vi "ResonanceAnalyzer.vi"() -> ()   [LabVIEW 2015]
uses:
  <vilib>/imath/engines/lvmath/Plug In/_Char/NIMS_CH_character datatype.ctl
  <vilib>/imath/engines/lvmath2/RunTimeEngine/Managers/WorkSpace/UID Generator.vi
  <vilib>/imath/engines/lvmath2/RunTimeEngine/RunTimeType/NIMS_RunTimeType_From StrictType (excl LVString).vi
  <instcachedir>/0/NIMS_RunTimeType_From StrictType (excl LVString)_EB1C38A9BC5048DA9ABDA8F781E54D21.lvgen/NIMS_RunTimeType_From StrictType (excl LVString)_EB1C38A9BC5048DA9ABDA8F781E54D21_000.vi
  <vilib>/imath/engines/lvmath2/RunTimeEngine/LocalVariableDefStatement/MC_LocalVariableDefStatement_Display.vi
  <vilib>/imath/engines/lvmath/Plug In/_Char/NIMS_CH_Character RV to String.vi
  <vilib>/imath/engines/lvmath2/RunTimeEngine/BuiltInFunctions/random/NIMS_random.vi
  <vilib>/imathl/engines/lvmath/Functions/Error Handling/Create Error.vi
  <vilib>/imath/engines/lvmath2/RunTimeEngine/NodeEndStatement/NIMS_NodeEndStatement_Get Scalar.vi
  <instcachedir>/0/NIMS_NodeEndStatement_Get Scalar_EFB59FDA1E10412DB5B4364F310E1970.lvgen/NIMS_NodeEndStatement_Get Scalar_EFB59FDA1E10412DB5B4364F310E1970_000.vi
  <vilib>/imath/engines/lvmath/Functions/Error Handling/MergeErrorsWrapper.vi
  <vilib>/imath/engines/lvmath2/RunTimeEngine/Managers/SymbolTable/Clear UID.vi
  <vilib>/imath/engines/lvmath2/RunTimeEngine/NodeEndStatement/NIMS_NodeEndStatement_Output.vi
  <instcachedir>/0/NIMS_NodeEndStatement_Output_53EC0D466D134D7ABD903AC30B43404B.lvgen/NIMS_NodeEndStatement_Output_53EC0D466D134D7ABD903AC30B43404B_001.vi
  <vilib>/imath/engines/lvmath2/RunTimeEngine/ErrorHandling/NIMS_Finalize Error.vi
  <vilib>/Utility/file.llb/Read Delimited Spreadsheet (DBL).vi
  <vilib>/imath/engines/lvmath2/RunTimeEngine/Managers/SymbolTable/NIMS_WorkSpace.lvlib
panel:
  out "XY Graph 2":cluster{"all rows":dbl[], "Array":dbl[]}(graph)
  out "Array 3":dbl[](array[numeric])
  out "Array 2":dbl[](array[numeric])
  out "Array":dbl[](array[numeric])
  out "XY Graph":cluster{"i":dbl[], "y":dbl[]}(graph)
  in  "Input Parameters":T1
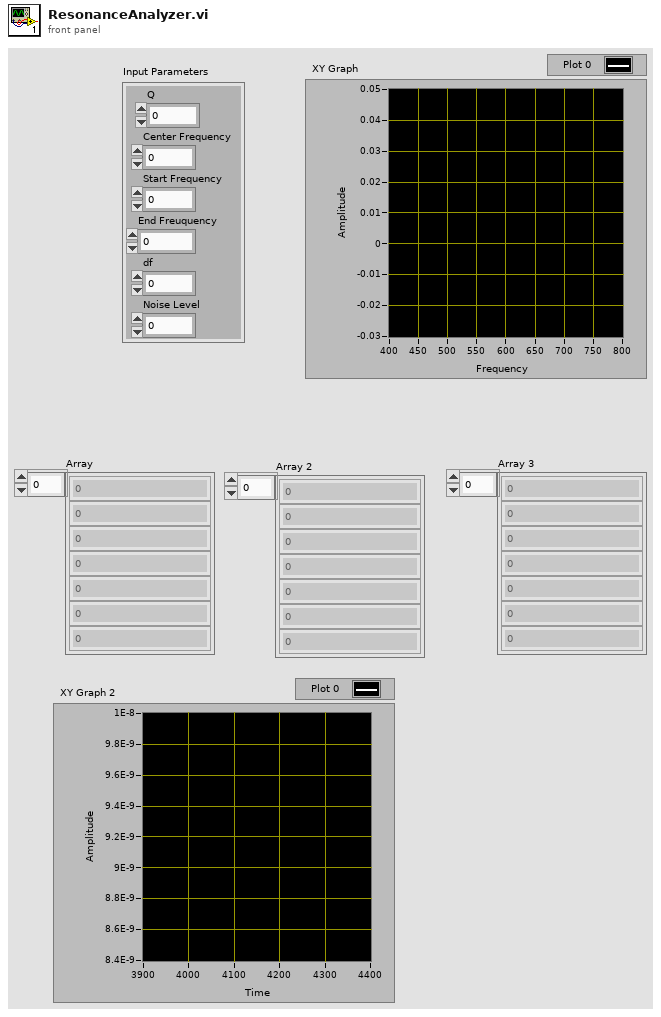
[diagram p1: front panel]
types:
  T1 = cluster{"Q":dbl, "Center Frequency ":dbl, "Start Frequency":dbl, "End Freuquency":dbl, "df":dbl, "Noise Level":dbl}
  T2 = typedef "NIMS_CH_character datatype.ctl" = cluster{"Numeric":u8}
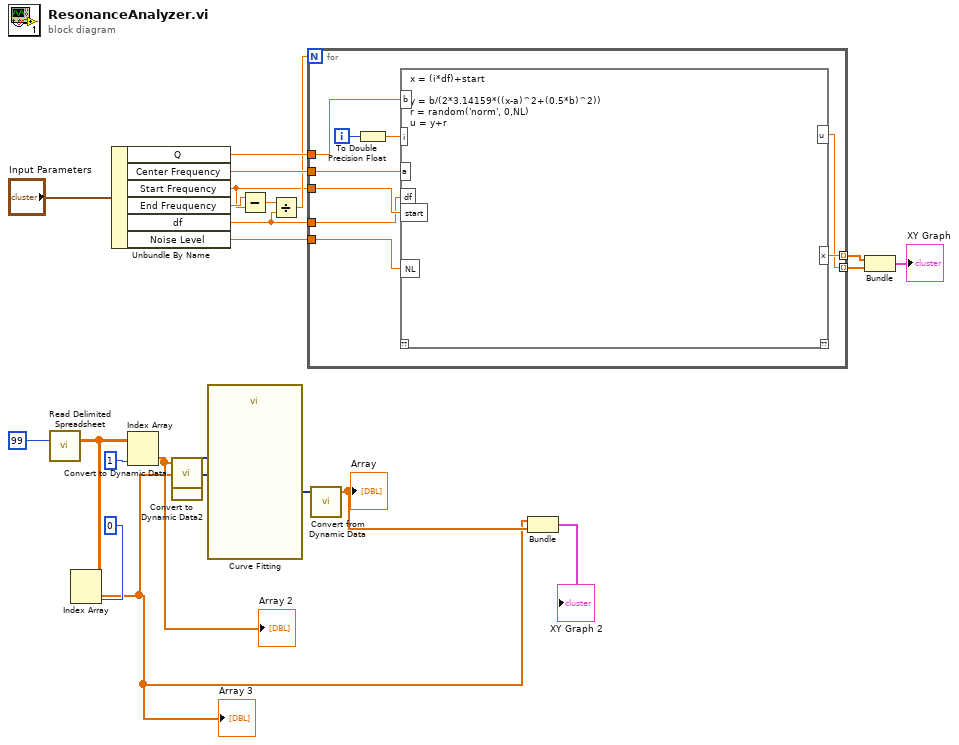
[diagram p0: block diagram]
diagram:
  n1 = call-poly <vilib>:"Read Delimited Spreadsheet.vi"("number of rows (all:-1)"=99) -> ("all rows"=w9:dbl[][])  [unwired: 9 in, 5 out]
  n2 = Index Array(array=w9, index (col)=0) -> (element=w2:dbl[])  [unwired: 1 in]
  "Array 3" <- w2
  n3 = Unbundle By Name("Input Parameters") -> ("Q"=w22:dbl, "Center Frequency"=w21:dbl, "Start Frequency"=w12:dbl, "End Freuquency"=w13:dbl, "df"=w16:dbl, "Noise Level"=w20:dbl)
  n4 = Index Array(array=w9, index (col)=1) -> (element=w6:dbl[])  [unwired: 1 in]
  "Array 2" <- w6
  n5 = call "Convert to Dynamic Data"("Array"=w6) -> ("Dynamic Data Type"=w5:dynamicdata)  [unwired: 3 in]
  n6 = call "Convert to Dynamic Data2"("Array"=w2) -> ("Dynamic Data Type"=w4:dynamicdata)  [unwired: 3 in]
  n7 = call "Curve Fitting"("Locations"=w4, "Signals"=w5) -> ("best fit"=w10:dynamicdata)  [unwired: 5 in, 4 out]
  n8 = Subtract(x=w13, y=w12) -> (x-y=w15:dbl)
  n9 = Divide(x=w15, y=w16) -> (x/y=w14:dbl)
  n10 = for {
    N: w14 -> [_]
    tunnel: [w32] -> w23 mode=indexing
    tunnel: [w31] -> w18 mode=indexing
    tunnel: w22 -> [w30]
    tunnel: w21 -> [w29]
    tunnel: w12 -> [w28]
    tunnel: w16 -> [w27]
    tunnel: w20 -> [w26]
    i -> [w25]
    n11 = To Double Precision Float(number=w25) -> (double precision float=w24:dbl)
    n12 = mathscript code="x = (i*df)+start\n\ny = b/(2*3.14159*((x-a)^2+(0.5*b)^2))\nr = random('norm', 0,NL)\nu = y+r"("b"=w30, "a"=w29, "df"=w27, "start"=w28, "NL"=w26, "i"=w24) -> ("u"=w31:dbl, "x"=w32:dbl)  [unwired: 1 in, 1 out]
  }
  n13 = call "Convert from Dynamic Data"("Dynamic Data Type"=w10) -> ("Array"=w3:dbl[])  [unwired: 3 in]
  "Array" <- w3
  n14 = Bundle("all rows"=w2, "Array"=w3) -> (→"XY Graph 2":cluster{"all rows":dbl[], "Array":dbl[]})  [unwired: 1 in]
  n15 = Bundle(w23, w18) -> (→"XY Graph":cluster{dbl[], dbl[]})  [unwired: 1 in]
